vi "HasNext.vi"(8 "error in (no error)":errorcluster, 11 "ArrayIterator":refnum<class "ArrayIterator.lvclass">) -> (0 "error out":errorcluster, 2 "HasNext(False)":bool, 3 "ArrayIterator out":refnum<class "ArrayIterator.lvclass">)   [LabVIEW 2015, in "ArrayIterator.lvclass"]
uses:
  ArrayIterator.lvclass
  BrowerComponent/BrowerComponent/BrowerComponent.lvclass
  ArrayIterator.lvclass/ArrayIterator.ctl
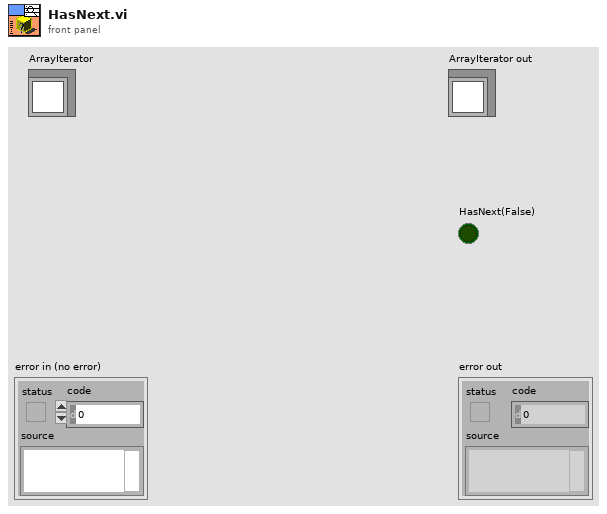
[diagram p1: front panel]
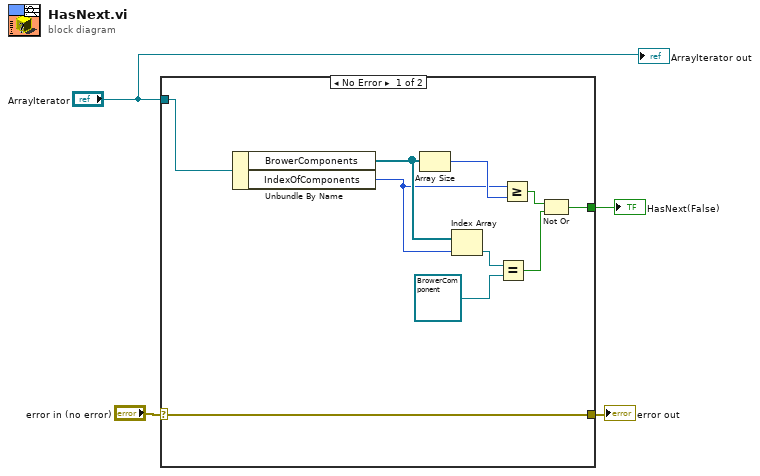
[diagram p0: block diagram]
diagram:
  n1 = case shown="No Error" "error in (no error)" {
    selector: "error in (no error)" -> [w6 w15]
    tunnel: "ArrayIterator" -> [w5 _]
    tunnel: [w9 _] -> w4
    tunnel: [w6 w15] -> w2
    frame No Error {
      n2 = Unbundle By Name(w5) -> ("BrowerComponents"=w8:refnum<class "BrowerComponent.lvclass">[], "IndexOfComponents"=w7:i32)
      n3 = Array Size(array=w8) -> (size(s)=w14:i32)
      n4 = Index Array(array=w8, index=w7) -> (element=w13:refnum<class "BrowerComponent.lvclass">)
      n5 = Equal?(x=w13, y=refnum<class "BrowerComponent.lvclass"> refnum) -> (x = y?=w10:bool)
      n6 = Greater Or Equal?(x=w7, y=w14) -> (x >= y?=w11:bool)
      n7 = Not Or(1:w10, 2:w11) -> (0:w9:bool)
    }
    frame Error {
    }
  }
  "error out" <- w2
  "HasNext(False)" <- w4
  "ArrayIterator out" <- "ArrayIterator"
